vi "UnregisterPublisherByType.vi"(7 "Event":refnum<class "Message Interface.lvclass">, 8 "error in (no error)":errorcluster, 11 "Message Broker Interface in":refnum<class "EDA Message Broker Interface Ref.lvclass">=refnum) -> (0 "error out":errorcluster, 3 "Message Broker Interface out":refnum<class "EDA Message Broker Interface Ref.lvclass">)   [LabVIEW 2016, in "Stream Mediator.lvlib" / "EDA Message Broker Interface Ref.lvclass"]
doc: "--\nCopyright © 2017 Composed SystemsI All rights reserved.\n\nAuthor: Jon McBee <jon.mcbee@composed.io>\n\nThis library is provided \"AS IS\" ,WITHOUT WARRANTIES OR\nCONDITIONS OF ANY KIND, either express or implied.\n\nComposed Systems -- composed.io\n\nStream 0.0.1.1\nJon McBee - Composed Systems\nCopyright (c) 2017, Composed Systems"
uses:
  <userlib>/Composed Systems/Stream/Mediator/Classes/EDA Message Broker Interface Ref/EDA Message Broker Interface Ref.lvclass
  C:/Program Files (x86)/National Instruments/LabVIEW 2016/user.lib/Composed Systems/Stream/Mediator/Classes/Message Broker Interface Ref/Message Broker Interface Ref.lvclass
  <userlib>/Composed Systems/Stream/Mediator/Classes/Message Interface/Message Interface.lvclass
  <userlib>/Composed Systems/Stream/Mediator/Classes/Message Broker/Message Broker.lvclass
  <userlib>/Composed Systems/Stream/Mediator/Classes/Message Broker Interface Ref/Message Broker Interface Ref.lvclass
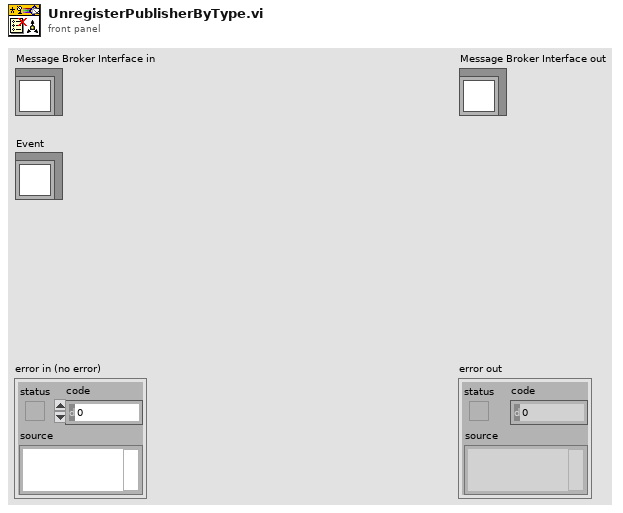
[diagram p1: front panel]
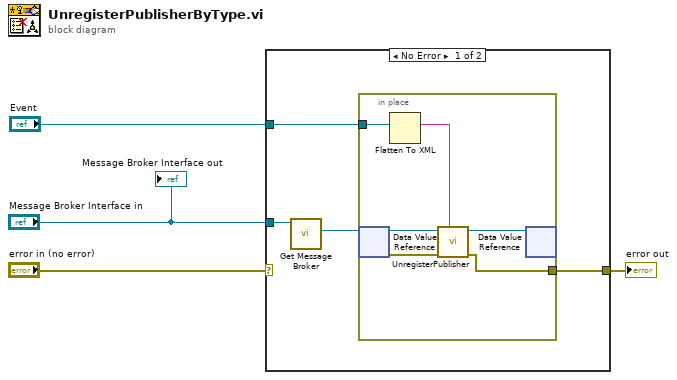
[diagram p0: block diagram]
diagram:
  n1 = case shown="No Error" "error in (no error)" {
    selector: "error in (no error)" -> [_ w15]
    tunnel: "Message Broker Interface in" -> [w8 _]
    tunnel: "Event" -> [w6 _]
    tunnel: [w5 w15] -> w1
    frame No Error {
      n2 = call <userlib>:"Get Message Broker.vi"("Message Broker Interface Ref in"=w8) -> ("Broker"=w7:refnum<data-value>)  [unwired: 8 in, 2 out]
      n3 = in-place {
        in-place-border: [w9] -> w5
        in-place-border: w6 -> [w11]
        n4 = in-place-dvr #1(w7) -> (w14:refnum<class "Message Broker.lvclass">, w12:errorcluster)
        n5 = Flatten To XML(anything=w11) -> (xml string=w10:string)
        n6 = call <userlib>:"UnregisterPublisher.vi"("Topic Name"=w10, "error in (no error)"=w12, "Message Broker in"=w14) -> ("error out"=w9:errorcluster, "Message Broker out"=w13:refnum<class "Message Broker.lvclass">)  [unwired: 7 in]
        n7 = in-place-dvr #1(w13) -> ()  [unwired: 2 out]
      }
    }
    frame Error {
    }
  }
  "error out" <- w1
  "Message Broker Interface out" <- "Message Broker Interface in"
